vi "Event based state machine.vi"() -> ()   [LabVIEW 2020]
uses:
  Enum type def.ctl
  <vilib>/Utility/miscctls.llb/LVPositionTypeDef.ctl
  Global variables.vi
panel:
  out "Saving...":bool
  out "?":u8(slide) scale=50.0..100.0
  out "?":u8(slide) scale=50.0..100.0
  out "?":u8(slide) scale=50.0..100.0
  in  "Blank Button 2":bool
  in  "ON/OFF 3":bool
  in  "ON/OFF 2":bool
  out "PROTON":bool
  in  "Third module U [V]":dbl(slide) scale=150000000000000.0..300000000000000.0 scale format="%#_6p"
  in  "Second module U [V]":dbl(slide) scale=150000000000000.0..300000000000000.0 scale format="%#_6p"
  out "Energy [J]":dbl
  out "Velocity [m/s]":dbl
  in  "Auto-Scalling":bool
  in  "First module U [V]":dbl(slide) scale=150000000000000.0..300000000000000.0 scale format="%#_6p"
  out "Module 3B":u16(ring)
  out "Module 3A":u16(ring)
  out "Module 2B":u16(ring)
  out "Module 2A":u16(ring)
  out "Module 1B":u16(ring)
  out "Module 1A":u16(ring)
  in  "stop program":bool
  in  "Image ring":u16(ring) items=["jpg", "bmp"]
  in  "Blank Button":bool
  out "stop":bool
  out "start":bool
  out "Velocity Diagram":T1(graph)
  in  "Reset":bool
  in  "Save data":bool
  in  "Write to file":u16(ring) items=["txt", "csv", "xls"]
  in  "Animation speed":dbl(slide) scale=0.001..0.05
  in  "Stop Button":bool
  in  "Start":bool
  in  "Save image":bool
  # "Data panel"
  # "Diagram"
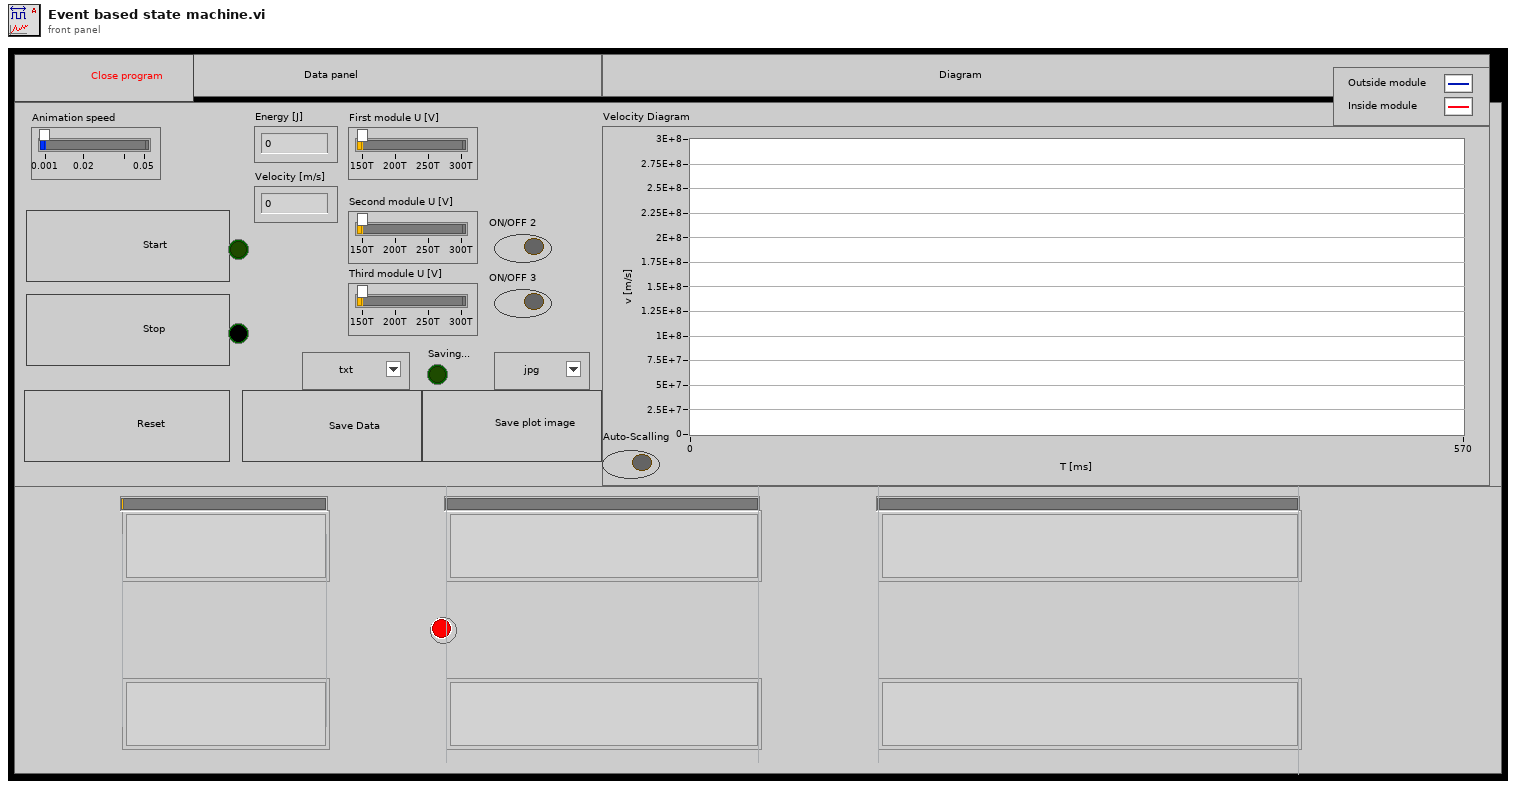
[diagram p1: front panel]
types:
  T1 = cluster{"Velocity (energy computed)":dbl, "Velocity (energy computed)":dbl}
  T2 = typedef "LVPositionTypeDef.ctl" = cluster{"Left":i32, "Top":i32}
  T3 = enum16{"Always On", "Always Off", "Off While Running"}
  T4 = typedef "Enum type def.ctl" = enum16{"Wait", "Start", "Stop", "Save data", "Reset", "Save image", "Mouse blockade", "Excess", "Erase"}
  T5 = enum8{"Enabled", "Disabled", "Disabled and Grayed Out"}
  T6 = typedef "imagedata.ctl" = cluster{"image type":i32, "image depth":i32, "image":u8[], "mask":u8[], "colors":u32[], "Rectangle":cluster{"left":i16, "top":i16, "right":i16, "bottom":i16}}
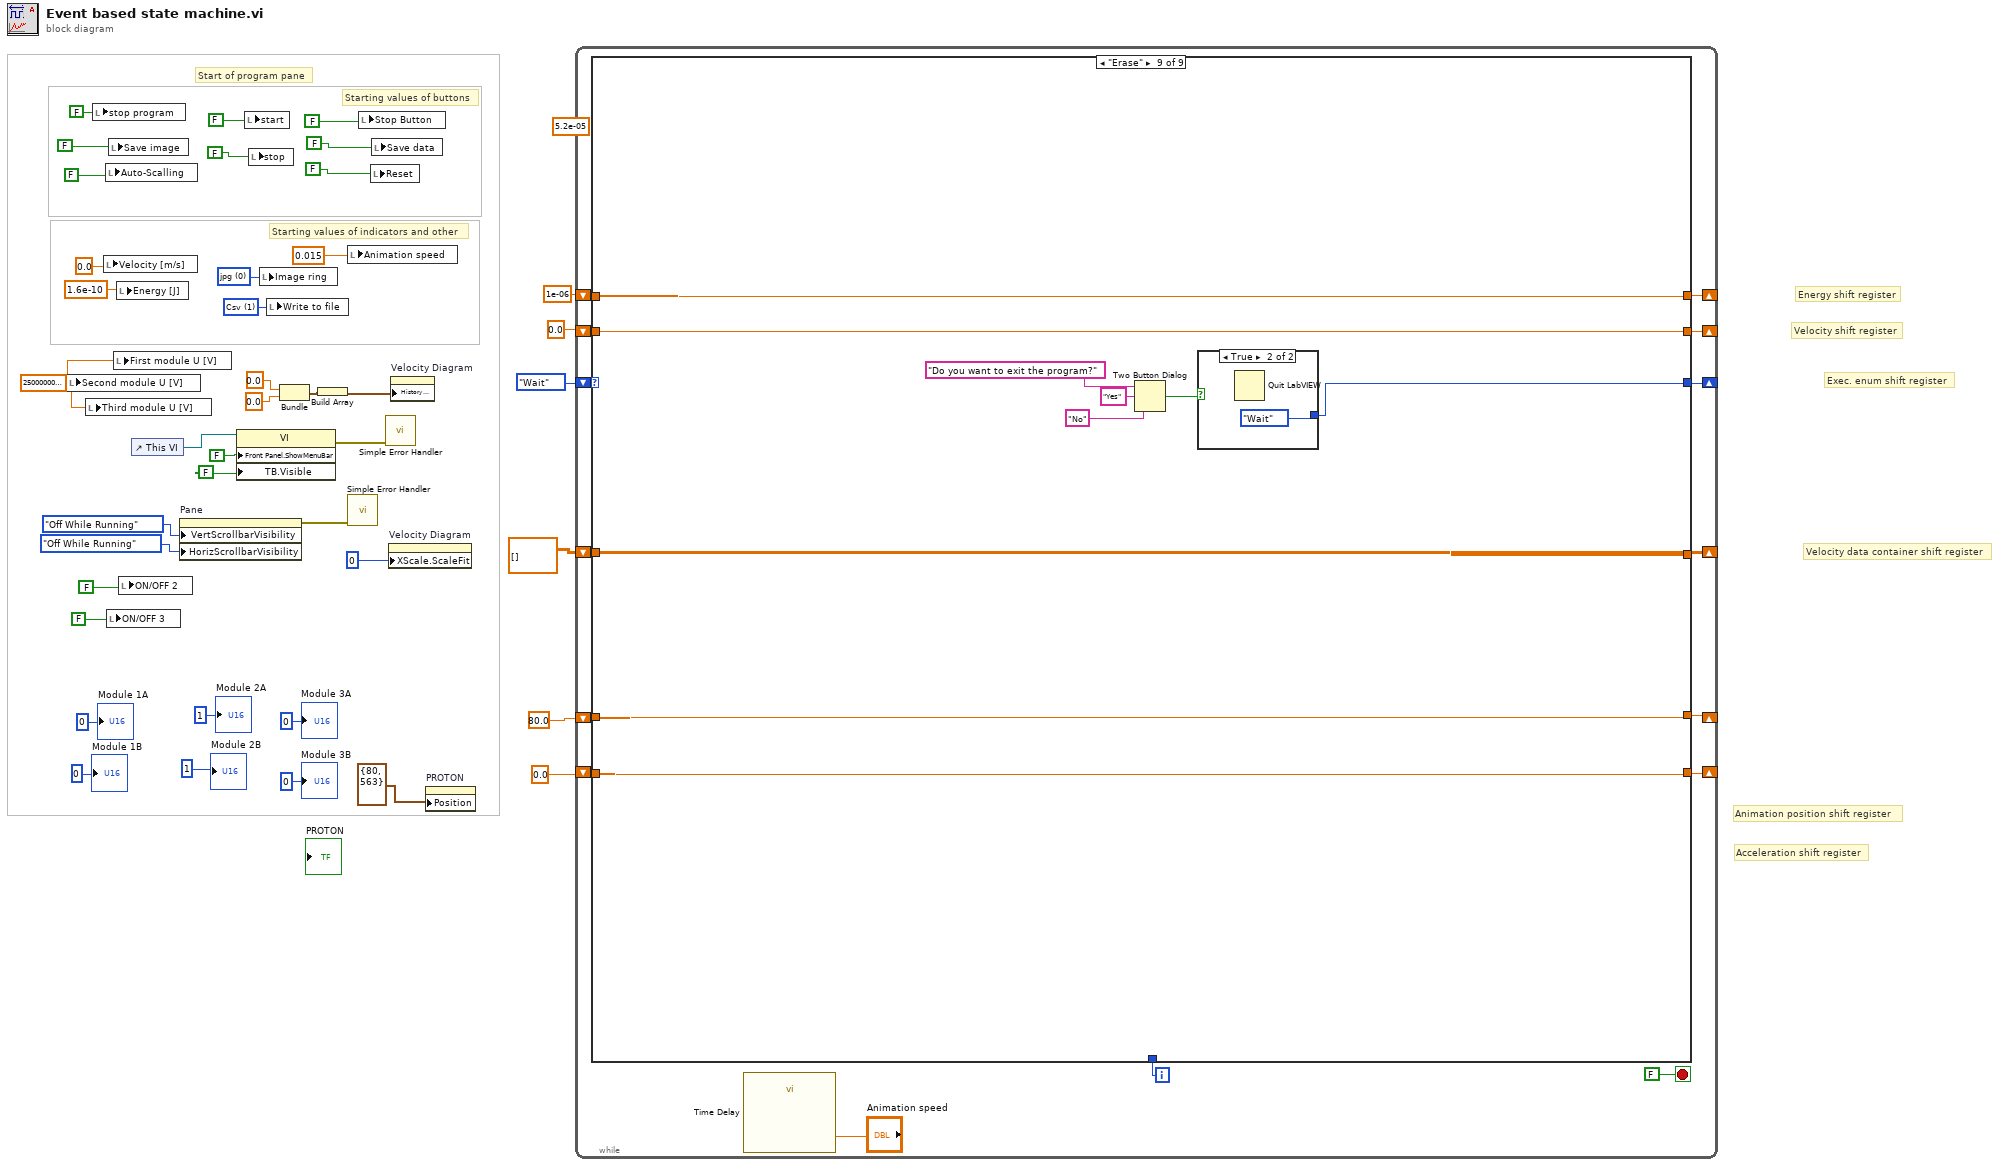
[diagram p0: block diagram]
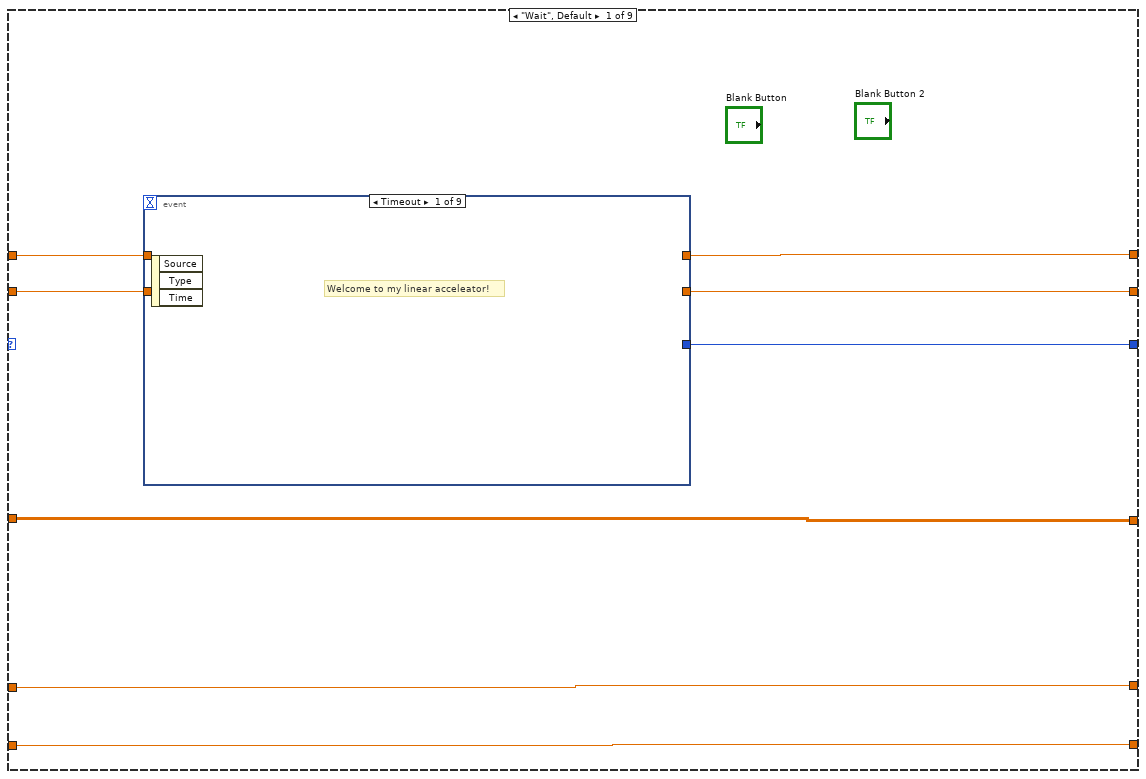
[diagram p2: hidden frame]
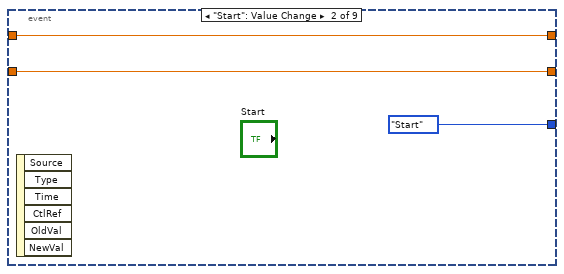
[diagram p3: hidden frame]
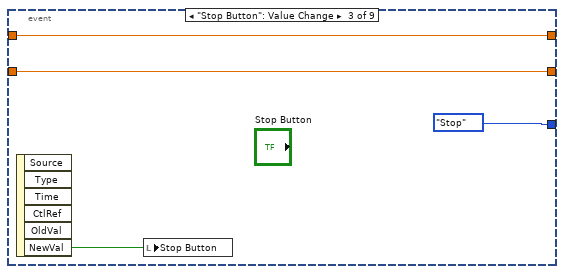
[diagram p4: hidden frame]
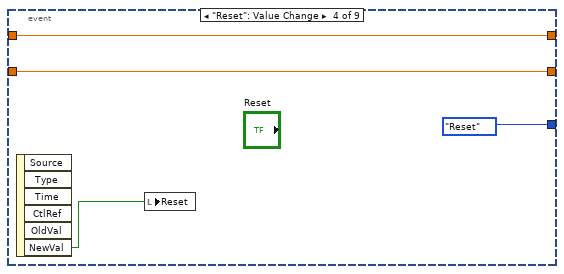
[diagram p5: hidden frame]
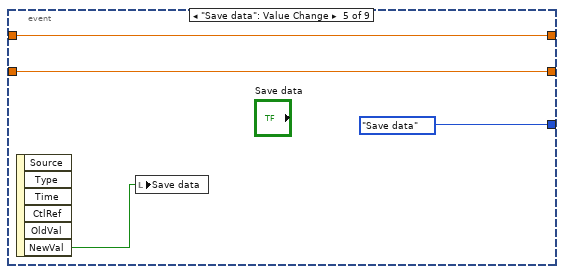
[diagram p6: hidden frame]
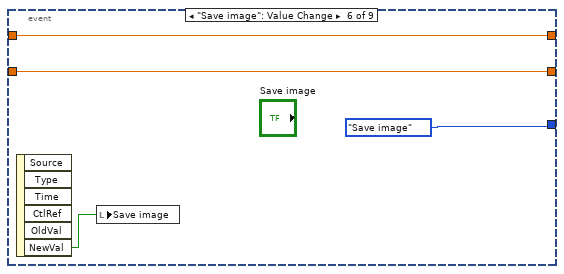
[diagram p7: hidden frame]
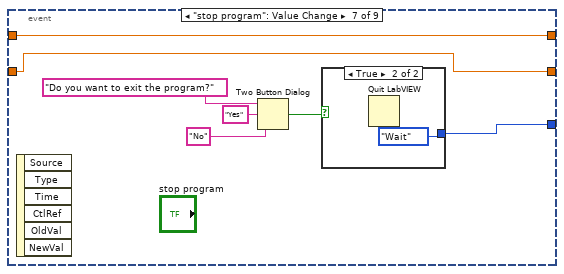
[diagram p8: hidden frame]
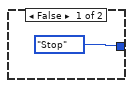
[diagram p9: hidden frame]
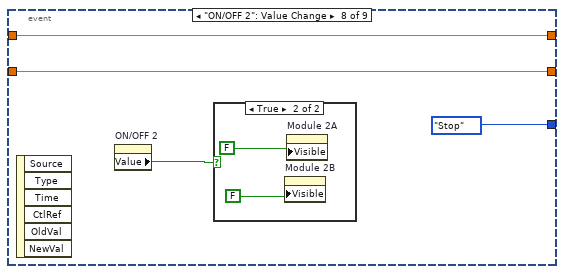
[diagram p10: hidden frame]
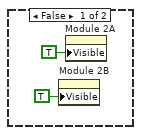
[diagram p11: hidden frame]
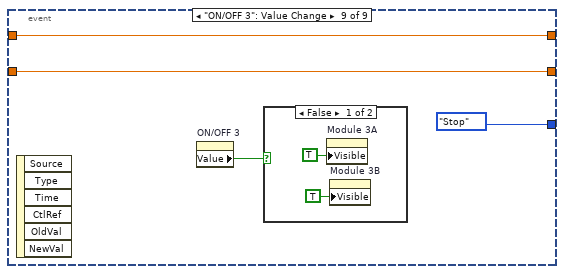
[diagram p12: hidden frame]
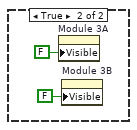
[diagram p13: hidden frame]
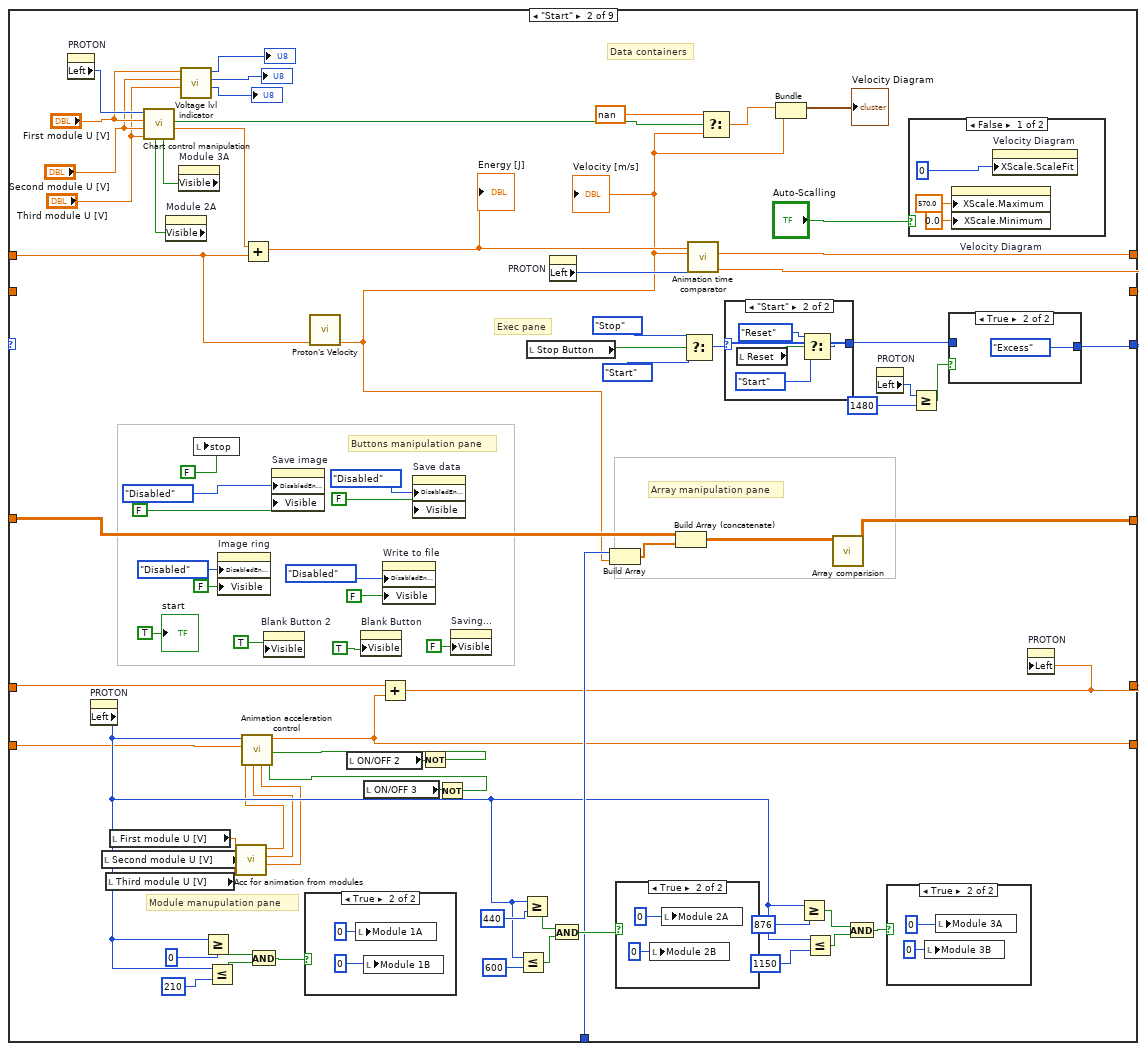
[diagram p14: hidden frame]
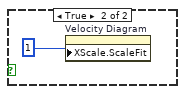
[diagram p16: hidden frame]
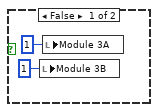
[diagram p17: hidden frame]
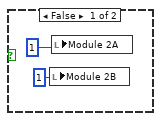
[diagram p18: hidden frame]
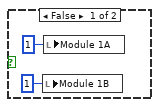
[diagram p19: hidden frame]
diagram:
  w6 = 250000000000000.0 ("2 module Voltage")
  w9 = u16 0 items=["jpg", "bmp"] ("Image ring")
  w10 = u16 1 items=["Txt", "Csv", "xls"] ("Write to file")
  (unwired) 5.2e-05
  # "Acceleration shift register"
  # "Animation position shift register"
  # "Starting values of indicators and other"
  # "Starting values of buttons"
  # "Start of program pane"
  # "Velocity data container shift register"
  # "Exec. enum shift register"
  # "Velocity shift register"
  # "Energy shift register"
  n1 = local write "Second module U [V]"(w6) -> ()
  n2 = local write "Third module U [V]"(w6) -> ()
  n3 = local write "stop program"(FALSE ("stop program")) -> ()
  n4 = local write "Velocity [m/s]"(0.0 ("Velocity [m/s]")) -> ()
  n5 = local write "Auto-Scalling"(FALSE ("Auto-Scalling")) -> ()
  n6 = local write "ON/OFF 3"(FALSE ("ON/OFF 3")) -> ()
  n7 = local write "Save image"(FALSE ("Save image")) -> ()
  n8 = local write "First module U [V]"(w6) -> ()
  n9 = local write "Energy [J]"(1.6e-10 ("Energy [J]")) -> ()
  n10 = local write "ON/OFF 2"(FALSE ("visibility of 2")) -> ()
  n11 = control-ref of="This VI"() -> (w35:refnum<vi>)
  n12 = property on="Pane" class="Pane"("VertScrollbarVisibility"=T3."Off While Running" ("Vertical Scrollbar Visibility"), "HorizScrollbarVisibility"=T3."Off While Running" ("Horizontal Scrollbar Visibility")) -> (error out=w37:errorcluster)  [unwired: 2 in, 1 out]
  n13 = property class="VI"(reference=w35, "Front Panel.ShowMenuBar"=FALSE ("Front Panel Window:Show Menu Bar"), "TB.Visible"=FALSE ("Tool Bar:Visible")) -> (error out=w36:errorcluster)  [unwired: 1 in, 1 out]
  n14 = local write "start"(FALSE ("start")) -> ()
  n15 = local write "stop"(FALSE ("stop")) -> ()
  n16 = local write "Image ring"(w9) -> ()
  n17 = local write "Write to file"(w10) -> ()
  n18 = Bundle(0.0, 0.0) -> (w38:cluster{dbl, dbl})  [unwired: 1 in]
  n19 = Build Array(w38) -> (w39:cluster{dbl, dbl}[])
  n20 = local write "Animation speed"(0.015 ("Animation speed")) -> ()
  n21 = call <vilib>:"Simple Error Handler.vi"("error in (no error)"=w37) -> ()  [unwired: 4 in, 5 out]
  n22 = local write "Stop Button"(FALSE) -> ()
  n23 = local write "Reset"(FALSE ("Reset")) -> ()
  n24 = local write "Save data"(FALSE ("Save data")) -> ()
  n25 = call <vilib>:"Simple Error Handler.vi"("error in (no error)"=w36) -> ()  [unwired: 4 in, 5 out]
  n26 = property on="Velocity Diagram" class="WFChart (strict)"("XScale.ScaleFit"=u8 0 ("X Scale.Scale Fit")) -> ()  [unwired: 2 in, 2 out]
  n27 = property on="Velocity Diagram" class="WFChart (strict)"("History Data"=w39) -> ()  [unwired: 2 in, 2 out]
  n28 = property on="PROTON" class="Bool (strict)"("Position"=T2 {"Left"=80, "Top"=563}) -> ()  [unwired: 2 in, 2 out]
  n29 = while {
    shift-right: [w53] -> _
    shift-left: Enum_type_def."Wait" -> [w56]
    shift-right: [w54] -> _
    shift-left: 1e-06 -> [w55]
    shift-right: [w52] -> _
    shift-left: 0.0 ("Velocity out") -> [w51]
    shift-right: [w48] -> _
    shift-left: dbl[][] [] -> [w49]
    shift-right: [w44] -> _
    shift-left: 80.0 -> [w45]
    shift-right: [w42] -> _
    shift-left: 0.0 ("Accelerated/no") -> [w43]
    i -> [w47]
    stop <- FALSE stop-if-true
    n30 = case shown="\"Erase\"" w56 {
      tunnel: [w64 w136 w210 Enum_type_def."Stop" Enum_type_def."Mouse blockade" Enum_type_def."Mouse blockade" Enum_type_def."Stop" Enum_type_def."Start" w331] -> w53
      tunnel: w55 -> [w63 w176 w243 _ w302 w313 w320 _ w340]
      tunnel: [w62 w141 w243 w291 w302 w313 w320 1e-06 w340] -> w54
      tunnel: [w60 w140 w242 w292 w301 w312 w319 0.0 w339] -> w52
      tunnel: w51 -> [w61 _ w242 w292 w301 w312 w319 _ w339]
      tunnel: w49 -> [w59 w179 w240 _ w300 w311 w317 _ w338]
      tunnel: [w59 w178 w240 dbl[][] [] w300 w311 w317 dbl[][] [] ("initialized array") w338] -> w48
      tunnel: w47 -> [_ w149 _ _ _ _ _ _ _]
      tunnel: w45 -> [w58 w168 w225 _ w298 w307 w316 _ w337]
      tunnel: [w58 w134 w225 w285 w298 w307 w316 80.0 ("Position:Left") w337] -> w44
      tunnel: w43 -> [w57 w132 w224 _ w297 w306 w315 _ w336]
      tunnel: [w57 w131 w224 0.0 ("Accelerated/no") w297 w306 w315 0.0 ("Accelerated/no") w336] -> w42
      frame "Wait", Default {
        n31 = event shown="[0] Timeout" {
          selector: _ -> [_ _ _ _ _ _ _ _ _]
          dyn-events: _ -> [_ _ _ _ _ _ _ _ _]
          timeout: _ -> [_ _ _ _ _ _ _ _ _]
          tunnel: [_ Enum_type_def."Start" Enum_type_def."Stop" Enum_type_def."Reset" Enum_type_def."Save data" Enum_type_def."Save image" w86 Enum_type_def."Stop" Enum_type_def."Stop"] -> w64
          tunnel: w63 -> [_ w67 w69 w73 w77 w81 w85 w94 w103]
          tunnel: [_ w67 w69 w73 w77 w81 w85 w94 w103] -> w62
          tunnel: w61 -> [_ w66 w68 w72 w76 w80 w84 w93 w102]
          tunnel: [_ w66 w68 w72 w76 w80 w84 w93 w102] -> w60
          event Timeout {
            # "Welcome to my linear acceleator!"
            n32 = event-data() -> ()  [unwired: 1 in, 3 out]
          }
          event "Start": Value Change {
            n33 = event-data() -> ()  [unwired: 1 in, 6 out]
          }
          event "Stop Button": Value Change {
            n34 = event-data() -> ("NewVal"=w71:bool)  [unwired: 1 in, 5 out]
            n35 = local write "Stop Button"(w71) -> ()
          }
          event "Reset": Value Change {
            n36 = event-data() -> ("NewVal"=w75:bool)  [unwired: 1 in, 5 out]
            n37 = local write "Reset"(w75) -> ()
          }
          event "Save data": Value Change {
            n38 = event-data() -> ("NewVal"=w79:bool)  [unwired: 1 in, 5 out]
            n39 = local write "Save data"(w79) -> ()
          }
          event "Save image": Value Change {
            n40 = event-data() -> ("NewVal"=w83:bool)  [unwired: 1 in, 5 out]
            n41 = local write "Save image"(w83) -> ()
          }
          event "stop program": Value Change {
            n42 = event-data() -> ()  [unwired: 1 in, 6 out]
            n43 = Two Button Dialog(message="Do you want to exit the program?", 1:"No" ("F button name (\"Cancel\")"), 2:"Yes" ("T button name (\"OK\")")) -> (T button?=w87:bool)
            n44 = case shown="True" w87 {
              tunnel: [Enum_type_def."Stop" Enum_type_def."Wait"] -> w86
              frame False {
              }
              frame True {
                n45 = Quit LabVIEW() -> ()  [unwired: 1 in]
              }
            }
          }
          event "ON/OFF 2": Value Change {
            n46 = event-data() -> ()  [unwired: 1 in, 6 out]
            n47 = property on="ON/OFF 2" class="Bool (strict)"() -> ("Value"=w95:bool)  [unwired: 2 in, 2 out]
            n48 = case shown="True" w95 {
              frame False {
                n49 = property on="Module 2B" class="Ring (strict)"("Visible"=TRUE) -> ()  [unwired: 2 in, 2 out]
                n50 = property on="Module 2A" class="Ring (strict)"("Visible"=TRUE) -> ()  [unwired: 2 in, 2 out]
              }
              frame True {
                n51 = property on="Module 2B" class="Ring (strict)"("Visible"=FALSE) -> ()  [unwired: 2 in, 2 out]
                n52 = property on="Module 2A" class="Ring (strict)"("Visible"=FALSE) -> ()  [unwired: 2 in, 2 out]
              }
            }
          }
          event "ON/OFF 3": Value Change {
            n53 = event-data() -> ()  [unwired: 1 in, 6 out]
            n54 = property on="ON/OFF 3" class="Bool (strict)"() -> ("Value"=w104:bool)  [unwired: 2 in, 2 out]
            n55 = case shown="False" w104 {
              frame False {
                n56 = property on="Module 3A" class="Ring (strict)"("Visible"=TRUE) -> ()  [unwired: 2 in, 2 out]
                n57 = property on="Module 3B" class="Ring (strict)"("Visible"=TRUE) -> ()  [unwired: 2 in, 2 out]
              }
              frame True {
                n58 = property on="Module 3A" class="Ring (strict)"("Visible"=FALSE) -> ()  [unwired: 2 in, 2 out]
                n59 = property on="Module 3B" class="Ring (strict)"("Visible"=FALSE) -> ()  [unwired: 2 in, 2 out]
              }
            }
          }
        }
      }
      frame "Start" {
        # "Module manupulation pane"
        # "Exec pane"
        # "Data containers"
        # "Buttons manipulation pane"
        # "Array manipulation pane"
        n60 = property on="PROTON" class="Bool (strict)"() -> ("Left"=w118:i32)  [unwired: 2 in, 2 out]
        n61 = property on="PROTON" class="Bool (strict)"() -> ("Left"=w133:i32)  [unwired: 2 in, 2 out]
        n62 = local read "Second module U [V]"() -> (w126:dbl)
        n63 = local read "Third module U [V]"() -> (w125:dbl)
        n64 = local read "First module U [V]"() -> (w127:dbl)
        n65 = property on="Module 2A" class="Ring (strict)"() -> ("Visible"=w119:bool)  [unwired: 2 in, 2 out]
        n66 = property on="Module 3A" class="Ring (strict)"() -> ("Visible"=w117:bool)  [unwired: 2 in, 2 out]
        n67 = call "Chart control manipulation.vi"("Visible 3"=w117, "Visible 2"=w119, "3rd module"="Third module U [V]", "2nd module"="Second module U [V]", "1st module"="First module U [V]", "Protons position"=w118) -> ("Energy from module"=w142:dbl, "Outside module?"=w116:bool)  [unwired: 4 in]
        n68 = call "Voltage lvl indicator.vi"("V3"="Third module U [V]", "V2"="Second module U [V]", "V1"="First module U [V]") -> (1:→"?":u8, 2:→"?":u8, 3:→"?":u8)  [unwired: 6 in]
        n69 = local write "stop"(FALSE ("stop")) -> ()
        n70 = Greater Or Equal?(x=w133, y=0) -> (x >= y?=w166:bool)
        n71 = Less Or Equal?(x=w133, y=210) -> (x <= y?=w165:bool)
        n72 = property on="Image ring" class="Ring (strict)"("DisabledEnum"=T5."Disabled" ("Disabled"), "Visible"=FALSE) -> ()  [unwired: 2 in, 2 out]
        n73 = call "Acc for animation from modules.vi"("Voltage 3 in"=w125, "Voltage 2 in"=w126, "Voltage 1 in"=w127) -> ("Acc 3 out"=w128:dbl, "Acc 2 out"=w129:dbl, "Acc 1 out"=w130:dbl)  [unwired: 6 in]
        n74 = Add(x=w142, y=w176) -> (x+y=w144:dbl)
        "Energy [J]" <- w144
        n75 = And(x=w166, y=w165) -> (x .and. y?=w150:bool)
        n76 = property on="Blank Button 2" class="Bool"("Visible"=TRUE) -> ()  [unwired: 2 in, 2 out]
        n77 = property on="Save image" class="Bool (strict)"("DisabledEnum"=T5."Disabled" ("Disabled"), "Visible"=FALSE) -> ()  [unwired: 2 in, 2 out]
        n78 = case shown="True" w150 {
          frame False {
            n79 = local write "Module 1B"(u16 1 ("Module 1B")) -> ()
            n80 = local write "Module 1A"(u16 1 ("Module 1A")) -> ()
          }
          frame True {
            n81 = local write "Module 1A"(u16 0 ("Module 1A")) -> ()
            n82 = local write "Module 1B"(u16 0 ("Module 1B")) -> ()
          }
        }
        n83 = call "Proton's Velocity.vi"("Starting kinetic energy"=w176) -> ("Velocity (energy computed)"=w143:dbl)  [unwired: 9 in, 1 out]
        "Velocity [m/s]" <- w143
        n84 = local read "ON/OFF 2"() -> (w123:bool)
        n85 = property on="Blank Button" class="Bool"("Visible"=TRUE) -> ()  [unwired: 2 in, 2 out]
        n86 = local read "ON/OFF 3"() -> (w121:bool)
        n87 = property on="Write to file" class="Ring (strict)"("DisabledEnum"=T5."Disabled" ("Disabled"), "Visible"=FALSE) -> ()  [unwired: 2 in, 2 out]
        n88 = property on="Save data" class="Bool (strict)"("DisabledEnum"=T5."Disabled" ("Disabled"), "Visible"=FALSE) -> ()  [unwired: 2 in, 2 out]
        n89 = Not(x=w123) -> (.not. x?=w122:bool)
        n90 = Not(x=w121) -> (.not. x?=w120:bool)
        n91 = call "Animation acceleration control.vi"("Visible 3 module"=w120, "Visible 2 module"=w122, "Volt 3"=w128, "Volt 2"=w129, "Volt 1"=w130, "Acc in"=w132, "Animation in"=w133) -> ("Acc out"=w131:dbl)  [unwired: 4 in]
        n92 = Add(x=w168, y=w131) -> (x+y=w134:dbl)
        n93 = property on="Saving..." class="Bool (strict)"("Visible"=FALSE) -> ()  [unwired: 2 in, 2 out]
        n94 = Less Or Equal?(x=w133, y=600) -> (x <= y?=w160:bool)
        n95 = Greater Or Equal?(x=w133, y=440) -> (x >= y?=w162:bool)
        n96 = local read "Stop Button"() -> (w186:bool)
        n97 = property on="PROTON" class="Bool (strict)"() -> ("Left"=w145:i32)  [unwired: 2 in, 2 out]
        n98 = And(x=w162, y=w160) -> (x .and. y?=w163:bool)
        n99 = Build Array(w149, w143) -> (w180:dbl[])
        n100 = case shown="True" w163 {
          frame False {
            n101 = local write "Module 2B"(u16 1 ("Module 2B")) -> ()
            n102 = local write "Module 2A"(u16 1 ("Module 2A")) -> ()
          }
          frame True {
            n103 = local write "Module 2B"(u16 0 ("Module 2B")) -> ()
            n104 = local write "Module 2A"(u16 0 ("Module 2A")) -> ()
          }
        }
        n105 = Build Array (concatenate)(w179, w180) -> (w177:dbl[][])
        n106 = Select(t=Enum_type_def."Stop", s=w186, f=Enum_type_def."Start") -> (s? t:f=w185:T4)
        n107 = call "Animation time comparator.vi"("Animation"=w145, "Velocity in"=w143, "Energy"=w144) -> ("Velocity out"=w140:dbl, "Energy out"=w141:dbl)  [unwired: 7 in]
        n108 = Select(t=nan, s=w116, f=w143) -> (s? t:f=w151:dbl)
        n109 = case shown="\"Start\"" w185 {
          selector: w185 -> [w205 _]
          tunnel: [w205 w208] -> w135
          frame "Stop", Default {
          }
          frame "Start" {
            n110 = local read "Reset"() -> (w209:bool)
            n111 = Select(t=Enum_type_def."Reset", s=w209, f=Enum_type_def."Start") -> (s? t:f=w208:T4)
          }
        }
        n112 = Bundle("Velocity (energy computed)"=w151, "Velocity (energy computed)"=w143) -> (→"Velocity Diagram":T1)  [unwired: 1 in]
        n113 = Greater Or Equal?(x=w133, y=876) -> (x >= y?=w157:bool)
        n114 = Less Or Equal?(x=w133, y=1150) -> (x <= y?=w156:bool)
        n115 = call "Array comparision.vi"("Array"=w177) -> ("initialized array"=w178:dbl[][])  [unwired: 10 in]
        n116 = And(x=w157, y=w156) -> (x .and. y?=w158:bool)
        n117 = property on="PROTON" class="Bool (strict)"() -> ("Left"=w139:i32)  [unwired: 2 in, 2 out]
        n118 = case shown="True" w158 {
          frame False {
            n119 = local write "Module 3B"(u16 1 ("Module 3B")) -> ()
            n120 = local write "Module 3A"(u16 1 ("Module 3A")) -> ()
          }
          frame True {
            n121 = local write "Module 3B"(u16 0 ("Module 3B")) -> ()
            n122 = local write "Module 3A"(u16 0 ("Module 3A")) -> ()
          }
        }
        n123 = case shown="False" "Auto-Scalling" {
          frame False {
            n124 = property on="Velocity Diagram" class="WFChart (strict)"("XScale.Maximum"=570.0 ("X Scale.Range:Maximum"), "XScale.Minimum"=0.0 ("X Scale.Range:Minimum")) -> ()  [unwired: 2 in, 2 out]
            n125 = property on="Velocity Diagram" class="WFChart (strict)"("XScale.ScaleFit"=u8 0 ("X Scale.Scale Fit")) -> ()  [unwired: 2 in, 2 out]
          }
          frame True {
            n126 = property on="Velocity Diagram" class="WFChart (strict)"("XScale.ScaleFit"=u8 1 ("X Scale.Scale Fit")) -> ()  [unwired: 2 in, 2 out]
          }
        }
        n127 = Greater Or Equal?(x=w139, y=1480) -> (x >= y?=w137:bool)
        n128 = case shown="True" w137 {
          tunnel: [w187 Enum_type_def."Excess"] -> w136
          tunnel: w135 -> [w187 _]
          frame False {
          }
          frame True {
          }
        }
        n129 = property on="PROTON" class="Bool (strict)"("Left"=w134) -> ()  [unwired: 2 in, 2 out]
        "start" <- TRUE ("start")
      }
      frame "Stop" {
        # "Exec pane"
        # "Buttons manipulation pane"
        n130 = local read "Second module U [V]"() -> (w219:dbl)
        n131 = local read "Third module U [V]"() -> (w218:dbl)
        n132 = local read "First module U [V]"() -> (w220:dbl)
        n133 = local read "Start"() -> (w241:bool)
        n134 = call "Voltage lvl indicator.vi"("V3"=w218, "V2"=w219, "V1"=w220) -> (1:w215:u8, 2:w216:u8, 3:w217:u8)  [unwired: 6 in]
        n135 = property on="Saving..." class="Bool (strict)"("Visible"=TRUE) -> ()  [unwired: 2 in, 2 out]
        n136 = Select(t=Enum_type_def."Start", s=w241, f=Enum_type_def."Stop") -> (s? t:f=w239:T4)
        n137 = property class="Slide (strict)"("Value"=w217) -> ()  [unwired: 2 in, 2 out]
        n138 = property class="Slide (strict)"("Value"=w215) -> ()  [unwired: 2 in, 2 out]
        n139 = property on="Save image" class="Bool (strict)"("DisabledEnum"=T5."Enabled" ("Disabled"), "Visible"=TRUE) -> ()  [unwired: 2 in, 2 out]
        n140 = property class="Slide (strict)"("Value"=w216) -> ()  [unwired: 2 in, 2 out]
        n141 = case shown="\"Stop\", Default" w239 {
          selector: w239 -> [w277 _]
          tunnel: [w277 w280] -> w236
          frame "Start" {
          }
          frame "Stop", Default {
            n142 = local read "Reset"() -> (w281:bool)
            n143 = Select(t=Enum_type_def."Reset", s=w281, f=Enum_type_def."Stop") -> (s? t:f=w280:T4)
          }
        }
        n144 = local write "start"(FALSE ("start")) -> ()
        n145 = case shown="False" "ON/OFF 3" {
          frame False {
            n146 = property on="Module 3A" class="Ring (strict)"("Visible"=TRUE) -> ()  [unwired: 2 in, 2 out]
            n147 = property on="Module 3B" class="Ring (strict)"("Visible"=TRUE) -> ()  [unwired: 2 in, 2 out]
            n148 = property class="Slide (strict)"("Visible"=TRUE) -> ()  [unwired: 2 in, 2 out]
          }
          frame True {
            n149 = property on="Module 3A" class="Ring (strict)"("Visible"=FALSE) -> ()  [unwired: 2 in, 2 out]
            n150 = property on="Module 3B" class="Ring (strict)"("Visible"=FALSE) -> ()  [unwired: 2 in, 2 out]
            n151 = property class="Slide (strict)"("Visible"=FALSE) -> ()  [unwired: 2 in, 2 out]
          }
        }
        n152 = case shown="\"Stop\", Default" w236 {
          selector: w236 -> [_ w275 w276]
          tunnel: [w273 w275 w276] -> w233
          frame "Stop", Default {
            n153 = local read "Save data"() -> (w274:bool)
            n154 = Select(t=Enum_type_def."Save data", s=w274, f=Enum_type_def."Stop") -> (s? t:f=w273:T4)
          }
          frame "Reset" {
          }
          frame "Start" {
          }
        }
        n155 = property on="Save data" class="Bool (strict)"("DisabledEnum"=T5."Enabled" ("Disabled"), "Visible"=TRUE) -> ()  [unwired: 2 in, 2 out]
        n156 = property on="Blank Button" class="Bool"("Visible"=FALSE) -> ()  [unwired: 2 in, 2 out]
        n157 = case shown="\"Stop\", Default" w233 {
          selector: w233 -> [_ w268 w269 w270]
          tunnel: [w266 w268 w269 w270] -> w211
          frame "Stop", Default {
            n158 = local read "Save image"() -> (w267:bool)
            n159 = Select(t=Enum_type_def."Save image", s=w267, f=Enum_type_def."Stop") -> (s? t:f=w266:T4)
          }
          frame "Start" {
          }
          frame "Save data" {
          }
          frame "Reset" {
          }
        }
        n160 = property on="Write to file" class="Ring (strict)"("DisabledEnum"=T5."Enabled" ("Disabled"), "Visible"=TRUE) -> ()  [unwired: 2 in, 2 out]
        n161 = case shown="False" "ON/OFF 2" {
          frame False {
            n162 = property on="Module 2A" class="Ring (strict)"("Visible"=TRUE) -> ()  [unwired: 2 in, 2 out]
            n163 = property on="Module 2B" class="Ring (strict)"("Visible"=TRUE) -> ()  [unwired: 2 in, 2 out]
            n164 = property class="Slide (strict)"("Visible"=TRUE) -> ()  [unwired: 2 in, 2 out]
          }
          frame True {
            n165 = property on="Module 2B" class="Ring (strict)"("Visible"=FALSE) -> ()  [unwired: 2 in, 2 out]
            n166 = property on="Module 2A" class="Ring (strict)"("Visible"=FALSE) -> ()  [unwired: 2 in, 2 out]
            n167 = property class="Slide (strict)"("Visible"=FALSE) -> ()  [unwired: 2 in, 2 out]
          }
        }
        n168 = case shown="\"Stop\", Default" w211 {
          selector: w211 -> [w244 w245 w246 _ w251]
          tunnel: [w244 w245 w246 w250 w251] -> w210
          frame "Reset" {
          }
          frame "Save image" {
          }
          frame "Save data" {
          }
          frame "Stop", Default {
            n169 = local read "stop program"() -> (w249:bool)
            n170 = Select(t=Enum_type_def."Erase", s=w249, f=Enum_type_def."Stop") -> (s? t:f=w250:T4)
          }
          frame "Start" {
          }
        }
        n171 = property on="Image ring" class="Ring (strict)"("DisabledEnum"=T5."Enabled" ("Disabled"), "Visible"=TRUE) -> ()  [unwired: 2 in, 2 out]
        n172 = property on="Blank Button 2" class="Bool"("Visible"=FALSE) -> ()  [unwired: 2 in, 2 out]
        "stop" <- TRUE ("stop")
      }
      frame "Reset" {
        w285 = 80 ("Position:Left")
        # "Starting values of meters, labels and proton"
        n173 = Bundle(0.0, 0.0) -> (w287:cluster{dbl, dbl})  [unwired: 1 in]
        n174 = local write "Velocity [m/s]"(0.0 ("Velocity [m/s]")) -> ()
        n175 = local write "Energy [J]"(1e-07 ("Energy [J]")) -> ()
        n176 = Build Array(w287) -> (w288:cluster{dbl, dbl}[])
        n177 = property on="Velocity Diagram" class="WFChart (strict)"("History Data"=w288) -> ()  [unwired: 2 in, 2 out]
        n178 = global read "Global variables.vi" "Starting energy"() -> (w291:dbl)
        n179 = property on="PROTON" class="Bool (strict)"("Left"=w285) -> ()  [unwired: 2 in, 2 out]
      }
      frame "Save data" {
        n180 = call "Save to file.vi"("2D array"=w300, "File type"="Write to file") -> ()  [unwired: 10 in]
        n181 = call <vilib>:"Set Busy.vi"("disable click? (T)"=FALSE) -> ()  [unwired: 9 in, 2 out]
        "Saving..." <- TRUE ("Saving...")
      }
      frame "Save image" {
        n182 = call <vilib>:"RGB to Color.vi"() -> ("Color"=w310:u32)  [unwired: 3 in]
        n183 = invoke on="Velocity Diagram" class="WFChart (strict)" method="Get Image"("bg color"=w310) -> ("image data"=w309:T6)  [unwired: 5 in, 5 out]
        n184 = call "Save image.vi"("Ring"="Image ring", "image data"=w309) -> ()  [unwired: 10 in]
        n185 = property on="Saving..." class="Bool (strict)"("Value"=TRUE ("Saving...")) -> ()  [unwired: 2 in, 2 out]
        n186 = call <vilib>:"Set Busy.vi"("disable click? (T)"=FALSE) -> ()  [unwired: 9 in, 2 out]
      }
      frame "Mouse blockade" {
        n187 = call <vilib>:"Unset Busy.vi"() -> ()  [unwired: 11 in, 1 out]
        n188 = property on="Saving..." class="Bool (strict)"("Value"=FALSE ("Saving...")) -> ()  [unwired: 2 in, 2 out]
      }
      frame "Excess" {
        # "Pane serves to restart animation effect, values of velocity, energy and diagram"
        n189 = Bundle(0.0, 0.0) -> (w324:cluster{dbl, dbl})  [unwired: 1 in]
        n190 = Build Array(w324) -> (w321:cluster{dbl, dbl}[])
        n191 = property on="Velocity Diagram" class="WFChart (strict)"("History Data"=w321) -> ()  [unwired: 2 in, 2 out]
      }
      frame "Erase" {
        n192 = Two Button Dialog(message="Do you want to exit the program?", 1:"No" ("F button name (\"Cancel\")"), 2:"Yes" ("T button name (\"OK\")")) -> (T button?=w332:bool)
        n193 = case shown="True" w332 {
          tunnel: [Enum_type_def."Stop" Enum_type_def."Wait"] -> w331
          frame False {
          }
          frame True {
            n194 = Quit LabVIEW() -> ()  [unwired: 1 in]
          }
        }
      }
    }
    n195 = call "Time Delay"("Delay Time (s)"="Animation speed") -> ()  [unwired: 10 in, 1 out]
  }
  "Module 1A" <- u16 0 ("Module 1A")
  "Module 1B" <- u16 0 ("Module 1B")
  "Module 2A" <- u16 1 ("Module 2A")
  "Module 2B" <- u16 1 ("Module 2B")
  "Module 3A" <- u16 0 ("Module 3A")
  "Module 3B" <- u16 0 ("Module 3B")
